vi "Knob Turn Data.vi"(7 "Switch":T1=enum."Position 1") -> (8 "Switch Message":string)   [LabVIEW 2018, in "TLMB.lvlib"]
uses:
  Projects/TLMB.lvlib
  type defs/Encoder Position.ctl
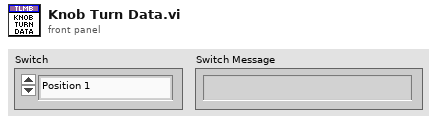
[diagram p1: front panel]
types:
  T1 = typedef "TLMB.lvlib/Encoder Position.ctl" = enum16{"Position 0", "Position 1", "Position 2", "Position 3", "Position 4", "Position 5", "Position 6", "Position 7", "Position 8", "Position 9", "Position 10", "Position 11", "Position 12", "Position 13", "Clear / Reset"}
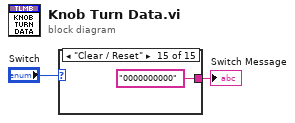
[diagram p0: block diagram]
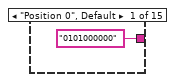
[diagram p2: hidden frame]
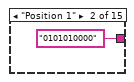
[diagram p3: hidden frame]
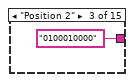
[diagram p4: hidden frame]
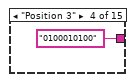
[diagram p5: hidden frame]
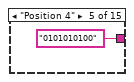
[diagram p6: hidden frame]
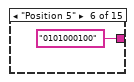
[diagram p7: hidden frame]
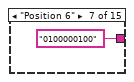
[diagram p8: hidden frame]
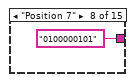
[diagram p9: hidden frame]
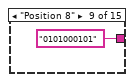
[diagram p10: hidden frame]
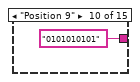
[diagram p11: hidden frame]
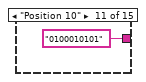
[diagram p12: hidden frame]
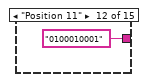
[diagram p13: hidden frame]
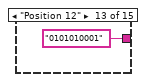
[diagram p14: hidden frame]
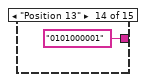
[diagram p15: hidden frame]
diagram:
  n1 = case shown="\"Clear / Reset\"" "Switch" {
    tunnel: ["0101000000" ("Message") "0101010000" ("Message") "0100010000" ("Message") "0100010100" ("Message") "0101010100" ("Message") "0101000100" ("Message") "0100000100" ("Message") "0100000101" ("Message") "0101000101" ("Message") "0101010101" ("Message") "0100010101" ("Message") "0100010001" ("Message") "0101010001" ("Message") "0101000001" ("Message") "0000000000" ("Message")] -> w1
    frame "Position 0", Default {
    }
    frame "Position 1" {
    }
    frame "Position 2" {
    }
    frame "Position 3" {
    }
    frame "Position 4" {
    }
    frame "Position 5" {
    }
    frame "Position 6" {
    }
    frame "Position 7" {
    }
    frame "Position 8" {
    }
    frame "Position 9" {
    }
    frame "Position 10" {
    }
    frame "Position 11" {
    }
    frame "Position 12" {
    }
    frame "Position 13" {
    }
    frame "Clear / Reset" {
    }
  }
  "Switch Message" <- w1
